vi "Build EthernetFrame (MAC).vi"(10 "MAC header":T1 {"EtherType" format="%04x"; "Src MAC" format="%02x"; "Dest MAC" format="%02x"}, 11 "Ethernet Frame In":u8[](array[numeric]) format="%.0x") -> (3 "Ethernet Frame Out":u8[](array[numeric]) format="%.0x")   [LabVIEW 2020, in "EthFrameManagement.lvlib"]
uses:
  EthFrameManagement.lvlib
  controls/ehternetFrame_type.ctl
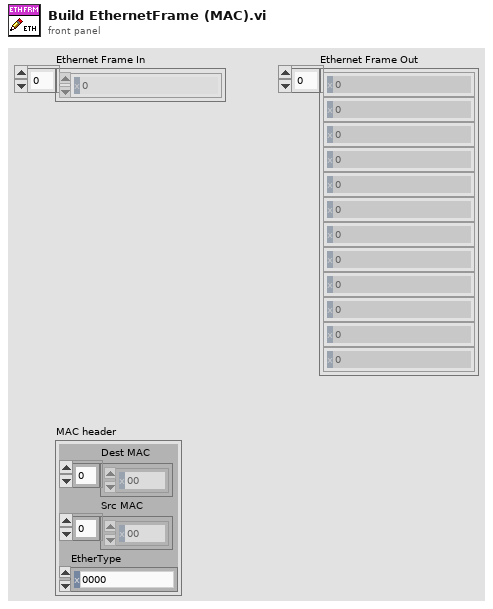
[diagram p1: front panel]
types:
  T1 = typedef "EthFrameManagement.lvlib/ehternetFrame_type.ctl" = cluster{"Dest MAC":u8[], "Src MAC":u8[], "EtherType":u16}
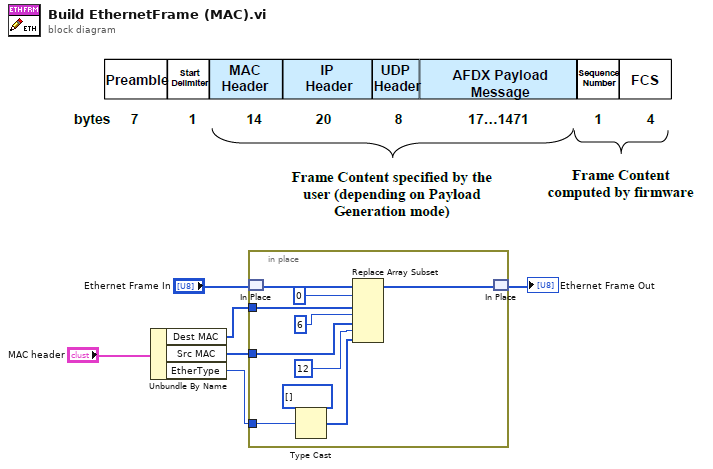
[diagram p0: block diagram]
diagram:
  n1 = Unbundle By Name("MAC header") -> ("Dest MAC"=w4:u8[], "Src MAC"=w3:u8[], "EtherType"=w2:u16)
  n2 = in-place {
    in-place-border: w4 -> [w14]
    in-place-border: w3 -> [w13]
    in-place-border: w2 -> [w9]
    n3 = in-place-match #1("Ethernet Frame In") -> (w16:u8[])
    n4 = Type Cast(type=u8[] [], x=w9) -> (*(type *) &x=w8:u8[])
    n5 = Replace Array Subset(array=w16, new element #1=w14, index #1=0 ("index"), new element #2=w13, index #2=6 ("index"), new element #3=w8, index #3=12 ("index")) -> (w11:u8[])
    n6 = in-place-match #1(w11) -> (→"Ethernet Frame Out":u8[])
  }
